vi "Update Message Converter VIs in Unary Method Call.vi"(6 "RPC Method Parameters":T1, 7 "Library":refnum<vi>, 8 "error in (no error)":errorcluster, 11 "VI in":refnum<vi>) -> (0 "error out":errorcluster, 3 "VI out":refnum<vi>)   [LabVIEW 2019, in "gRPC Template Creation Utility.lvlib"]
uses:
  gRPC Template Creation Utility.lvlib
  TypeDefs/RPC Method Parameters.ctl
  OneOf Constants/OneOfConstantsEnum.ctl
panel:
  out "Library out":refnum<vi>
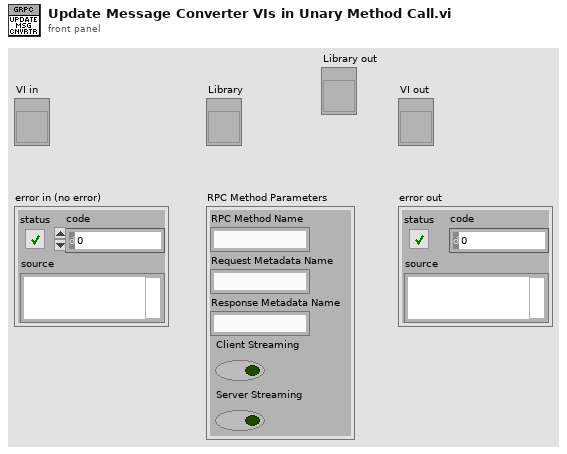
[diagram p1: front panel]
types:
  T1 = typedef "gRPC Template Creation Utility.lvlib/RPC Method Parameters.ctl" = cluster{"RPC Method Name":string, "Request Metadata Name":string, "Response Metadata Name":string, "Client Streaming":bool, "Server Streaming":bool}
  T2 = typedef "gRPC Template Creation Utility.lvlib/OneOfConstantsEnum.ctl" = enum16{"FlatToRichVIPrefix", "RichToFlatVIPrefix", "FlatTypeDefSuffix", ""}
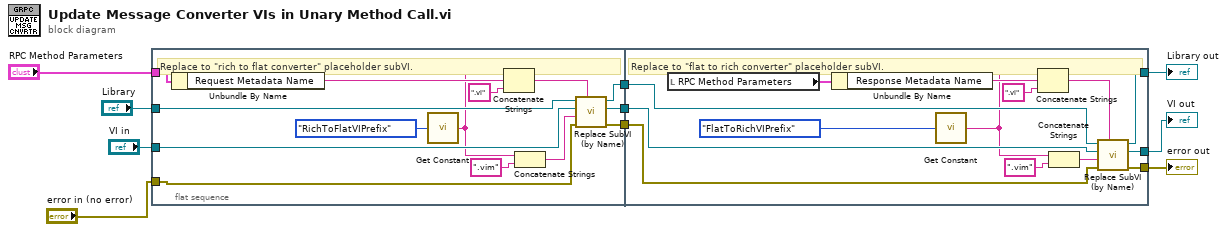
[diagram p0: block diagram]
diagram:
  n1 = flat-sequence {
    tunnel: "RPC Method Parameters" -> [w23]
    tunnel: "error in (no error)" -> [w16]
    tunnel: "Library" -> [w15]
    tunnel: "VI in" -> [w14]
    tunnel: [w19] -> w6
    tunnel: [w18] -> w5
    tunnel: [w17] -> w4
    tunnel: w6 -> [w36]
    tunnel: w5 -> [w37]
    tunnel: w4 -> [w38]
    tunnel: [w35] -> w3
    tunnel: [w34] -> w2
    tunnel: [w33] -> w1
    frame #0 {
      # "Replace to \"rich to flat converter\" placeholder subVI."
      n2 = Unbundle By Name(w23) -> ("Request Metadata Name"=w22:string)
      n3 = call "Get Constant.vi"("Selection"=OneOfConstantsEnum."RichToFlatVIPrefix") -> ("String"=w11:string)
      n4 = Concatenate Strings(w11, w22, ".vi" ("string")) -> (w21:string)
      n5 = Concatenate Strings(w11, ".vim" ("SubVI Name")) -> (w12:string)
      n6 = call "Replace SubVI (by Name).vi"("SubVI to replace with"=w21, "error in (no error)"=w16, "SubVI being replaced"=w12, "VI in"=w14, "Library in"=w15) -> ("error out"=w17:errorcluster, "VI out"=w18:refnum<vi>, "Library out"=w19:refnum<vi>)  [unwired: 4 in]
    }
    frame #1 {
      # "Replace to \"flat to rich converter\" placeholder subVI."
      n7 = local read "RPC Method Parameters"() -> (w31:T1)
      n8 = Unbundle By Name(w31) -> ("Response Metadata Name"=w32:string)
      n9 = call "Get Constant.vi"("Selection"=OneOfConstantsEnum."FlatToRichVIPrefix") -> ("String"=w25:string)
      n10 = Concatenate Strings(w25, w32, ".vi" ("string")) -> (w29:string)
      n11 = Concatenate Strings(w25, ".vim" ("SubVI Name")) -> (w26:string)
      n12 = call "Replace SubVI (by Name).vi"("SubVI to replace with"=w29, "error in (no error)"=w38, "SubVI being replaced"=w26, "VI in"=w37, "Library in"=w36) -> ("error out"=w35:errorcluster, "VI out"=w34:refnum<vi>, "Library out"=w33:refnum<vi>)  [unwired: 4 in]
    }
  }
  "error out" <- w3
  "VI out" <- w2
  "Library out" <- w1
